vi "ANC300_Open.vi"(0 "ANC300 Communication Port In":refnum<visa-resource-name>, 1 "IP":string="10.10.1.128", 4 "milliseconds to wait":u32=200, 8 "popup when problem":bool) -> (14 "ANC300 Communication Port Out":refnum<visa-resource-name>, 15 "connection ID out":refnum<k5>, 16 "OpeningData_1":string, 17 "OpeningData_2":string, 19 "error out":T1)   [LabVIEW 2022 SP3]
uses:
  <vilib>/Instr/_visa.llb/VISA Configure Serial Port (Instr).vi
panel:
  out "error out 2":errorcluster
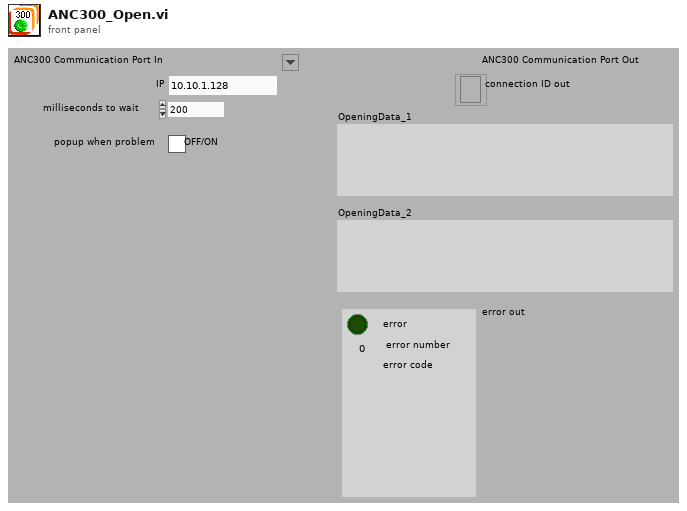
[diagram p1: front panel]
types:
  T1 = cluster{"error ":bool, "error number":i32, "error code":string}
  T2 = cluster{"error":bool, "error number":i32, "error code":string}
  T3 = enum16{"Standard", "Buffered", "CRLF", "Immediate"}
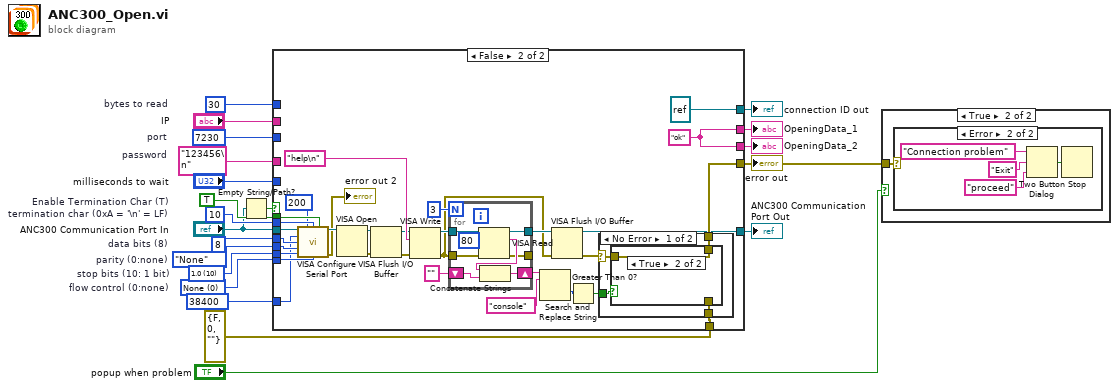
[diagram p0: block diagram]
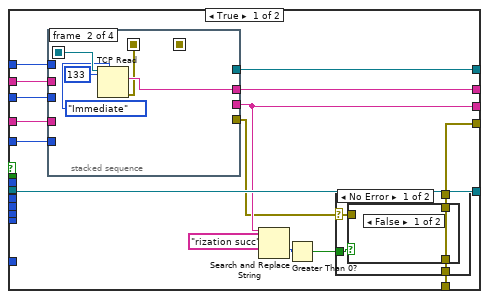
[diagram p4: hidden frame]
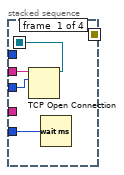
[diagram p7: hidden frame]
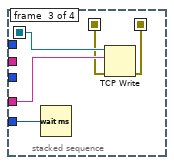
[diagram p8: hidden frame]
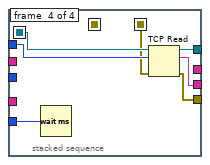
[diagram p9: hidden frame]
diagram:
  w8 = u8 10  # termination char (0xA = '\n' = LF)
  w9 = TRUE  # Enable Termination Char (T)
  w10 = u16 8  # data bits (8)
  w11 = enum16{"None", "Odd", "Even", "Mark", "Space"}."None"  # parity (0:none)
  w12 = u16 10 items=["1.0"=10, "1.5"=15, "2.0"=20]  # stop bits (10: 1 bit)
  w13 = u16 0 items=["None"=0, "XON/XOFF"=1, "RTS/CTS"=2, "DTR/DSR"=4, "XON/XOFF & RTS/CTS"=3, "XON/XOFF & DTR/DSR"=5]  # flow control (0:none)
  w16 = 30  # bytes to read
  w19 = "123456\n"  # password
  w20 = u16 7230  # port
  n1 = Empty String/Path?(string/path="ANC300 Communication Port In") -> (empty?=w5:bool)
  n2 = case shown="False" w5 {
    tunnel: "IP" -> [w36 _]
    tunnel: w20 -> [w35 _]
    tunnel: w19 -> [w34 _]
    tunnel: "milliseconds to wait" -> [w33 _]
    tunnel: [w32 w86] -> w17
    tunnel: w16 -> [w31 _]
    tunnel: [w30 refnum<k5> refnum ("connection ID")] -> w15
    tunnel: [w26 w86] -> w14
    tunnel: [w22 w75] -> w2
    tunnel: "ANC300 Communication Port In" -> [w29 w95]
    tunnel: w13 -> [_ w94]
    tunnel: w12 -> [_ w93]
    tunnel: w11 -> [_ w92]
    tunnel: w10 -> [_ w91]
    tunnel: w9 -> [_ w89]
    tunnel: w8 -> [_ w88]
    tunnel: [w29 w72] -> w7
    tunnel: u32 38400 ("baud rate (9600)") -> [_ w85]
    tunnel: T2 {"error"=FALSE, "error number"=0, "error code"=""} ("error out 3") -> [w23 w74]
    frame True {
      n3 = stacked-sequence {
        seq-local: [w47 _ _ _] -> [_ w52 w57 w64]
        seq-local: [_ w49 _ _] -> [_ _ w54 _]
        seq-local: [_ _ w53 _] -> [_ _ _ w59]
        tunnel: w36 -> [w46 _ _ _]
        tunnel: w35 -> [w45 _ _ _]
        tunnel: w34 -> [_ _ w56 _]
        tunnel: w33 -> [w44 _ w55 w60]
        tunnel: [_ w50 _ _] -> w32
        tunnel: w31 -> [_ _ _ w63]
        tunnel: [_ _ _ w62] -> w30
        tunnel: [_ _ _ w61] -> w26
        tunnel: [_ _ _ w58] -> w24
        frame #0 {
          n4 = TCP Open Connection(address=w46, remote port or service name=w45) -> (connection ID=w47:refnum<k5>)  [unwired: 3 in, 1 out]
          n5 = Wait (ms)(milliseconds to wait=w44) -> ()  [unwired: 1 out]
        }
        frame #1 {
          n6 = TCP Read(connection ID=w52, bytes to read=133, 7:T3."Immediate" ("mode (standard)")) -> (data out=w50:string, error out=w49:errorcluster)  [unwired: 2 in, 1 out]
        }
        frame #2 {
          n7 = Wait (ms)(milliseconds to wait=w55) -> ()  [unwired: 1 out]
          n8 = TCP Write(connection ID=w57, data in=w56, error in (no error)=w54) -> (error out=w53:errorcluster)  [unwired: 1 in, 2 out]
        }
        frame #3 {
          n9 = Wait (ms)(milliseconds to wait=w60) -> ()  [unwired: 1 out]
          n10 = TCP Read(connection ID=w64, bytes to read=w63, error in (no error)=w59) -> (connection ID out=w62:refnum<k5>, data out=w61:string, error out=w58:errorcluster)  [unwired: 2 in]
        }
      }
      n11 = Search and Replace String(input string=w26, search string="rization succ") -> (offset past replacement=w28:i32)  [unwired: 6 in, 3 out]
      n12 = Greater Than 0?(x=w28) -> (x > 0?=w27:bool)
      n13 = case shown="No Error" w24 {
        selector: w24 -> [w39 w43]
        tunnel: w27 -> [w40 _]
        tunnel: [w38 w43] -> w22
        tunnel: w23 -> [w37 _]
        frame No Error {
          n14 = case shown="False" w40 {
            tunnel: w39 -> [_ w42]
            tunnel: [w41 w42] -> w38
            tunnel: w37 -> [w41 _]
            frame False {
            }
            frame True {
            }
          }
        }
        frame Error {
        }
      }
    }
    frame False {
      w86 = "ok"
      n15 = call-poly "VISA Configure Serial Port"("VISA resource name"=w95, "timeout (10sec)"=u32 200, "termination char\n(0xA = '\\n' = LF)"=w88, "Enable Termination\nChar (T)"=w89, "baud rate (9600)"=w85, "data bits (8)"=w91, "parity (0:none)"=w92, "stop bits (10: 1 bit)"=w93, "flow control (0:none)"=w94) -> ("VISA resource name out"=w90:refnum<visa-resource-name>, "error out"=→"error out 2":errorcluster)  [unwired: 5 in]
      n16 = VISA Open(VISA resource name=w90) -> (VISA resource name=w67:refnum<visa-resource-name>, error out=w70:errorcluster)  [unwired: 4 in]
      n17 = VISA Flush I/O Buffer(VISA resource name=w67, error in (no error)=w70) -> (VISA resource name out=w68:refnum<visa-resource-name>, error out=w69:errorcluster)  [unwired: 1 in]
      n18 = VISA Write(VISA resource name=w68, write buffer="help\n", error in (no error)=w69) -> (VISA resource name out=w83:refnum<visa-resource-name>, error out=w65:errorcluster)  [unwired: 1 out]
      n19 = for {
        N: 3 -> [_]
        tunnel: w83 -> [w110]
        tunnel: w65 -> [w109]
        shift-right: [w106] -> w78
        shift-left: "" -> [w105]
        tunnel: [w104] -> _
        tunnel: [w103] -> w73
        n20 = VISA Read(VISA resource name=w110, byte count=u32 80, error in (no error)=w109) -> (VISA resource name out=w103:refnum<visa-resource-name>, read buffer=w107:string, error out=w104:errorcluster)  [unwired: 1 out]
        n21 = Concatenate Strings(w107, w105) -> (w106:string)
      }
      n22 = Search and Replace String(input string=w78, search string="console") -> (offset past replacement=w79:i32)  [unwired: 6 in, 3 out]
      n23 = VISA Flush I/O Buffer(VISA resource name=w73, error in (no error)=w65) -> (VISA resource name out=w72:refnum<visa-resource-name>, error out=w66:errorcluster)  [unwired: 1 in]
      n24 = Greater Than 0?(x=w79) -> (x > 0?=w76:bool)
      n25 = case shown="No Error" w66 {
        selector: w66 -> [w98 w102]
        tunnel: w76 -> [w99 _]
        tunnel: [w97 w102] -> w75
        tunnel: w74 -> [w96 _]
        frame No Error {
          n26 = case shown="True" w99 {
            tunnel: w98 -> [_ w101]
            tunnel: [w100 w101] -> w97
            tunnel: w96 -> [w100 _]
            frame False {
            }
            frame True {
            }
          }
        }
        frame Error {
        }
      }
    }
  }
  "error out" <- w2
  "OpeningData_1" <- w17
  "connection ID out" <- w15
  "OpeningData_2" <- w14
  "ANC300 Communication Port Out" <- w7
  n27 = case shown="True" "popup when problem" {
    tunnel: w2 -> [_ w111]
    frame False {
    }
    frame True {
      n28 = case shown="Error" w111 {
        frame No Error {
        }
        frame Error {
          n29 = Two Button Dialog(message="Connection problem", 1:"proceed" ("F button name (\"Cancel\")"), 2:"Exit" ("T button name (\"OK\")")) -> (T button?=w112:bool)
          n30 = Stop(stop? (T)=w112) -> ()
        }
      }
    }
  }
